vi "AcurrDataIn.vi"(0 "AMP":dbl, 1 "Max":dbl, 2 "Period":dbl, 3 "通道":u16(ring) items=["CH1", "CH2", "CH3", "CH4", "CH5", "CH6", "CH7", "CH8", "CH9", "CH10"], 5 "RMS":dbl, 7 "Min":dbl, 9 "Vpkpk":dbl, 11 "error in (no error)":errorcluster, 12 "FREQ":dbl, 13 "温度":dbl, 14 "测试类型":string) -> (15 "error out":errorcluster)   [LabVIEW 2014]
uses:
  <vilib>/addons/database/Connection.llb/DB Tools Open Connec (String).vi
  <vilib>/addons/database/Connection.llb/Conn Execute.vi
  <vilib>/addons/database/Recordset.llb/Rec Destroy - Connection.vi
  <vilib>/addons/database/NI_Database_API.lvlib
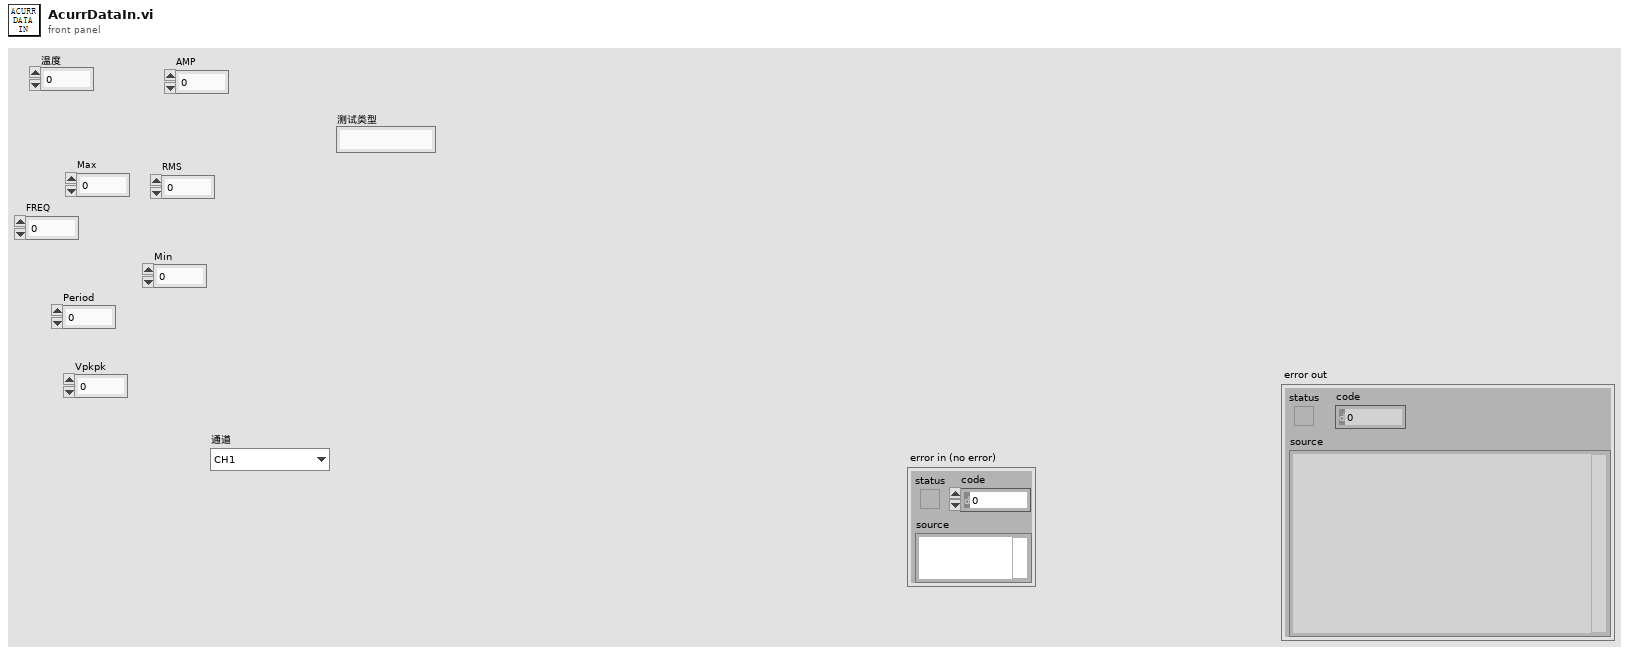
[diagram p1: front panel]
types:
  T1 = typedef "NI_Database_API.lvlib/Conn ObjectReference.ctl" = refnum<k1>
  T2 = typedef "NI_Database_API.lvlib/Rec ObjectReference.ctl" = refnum<k1>
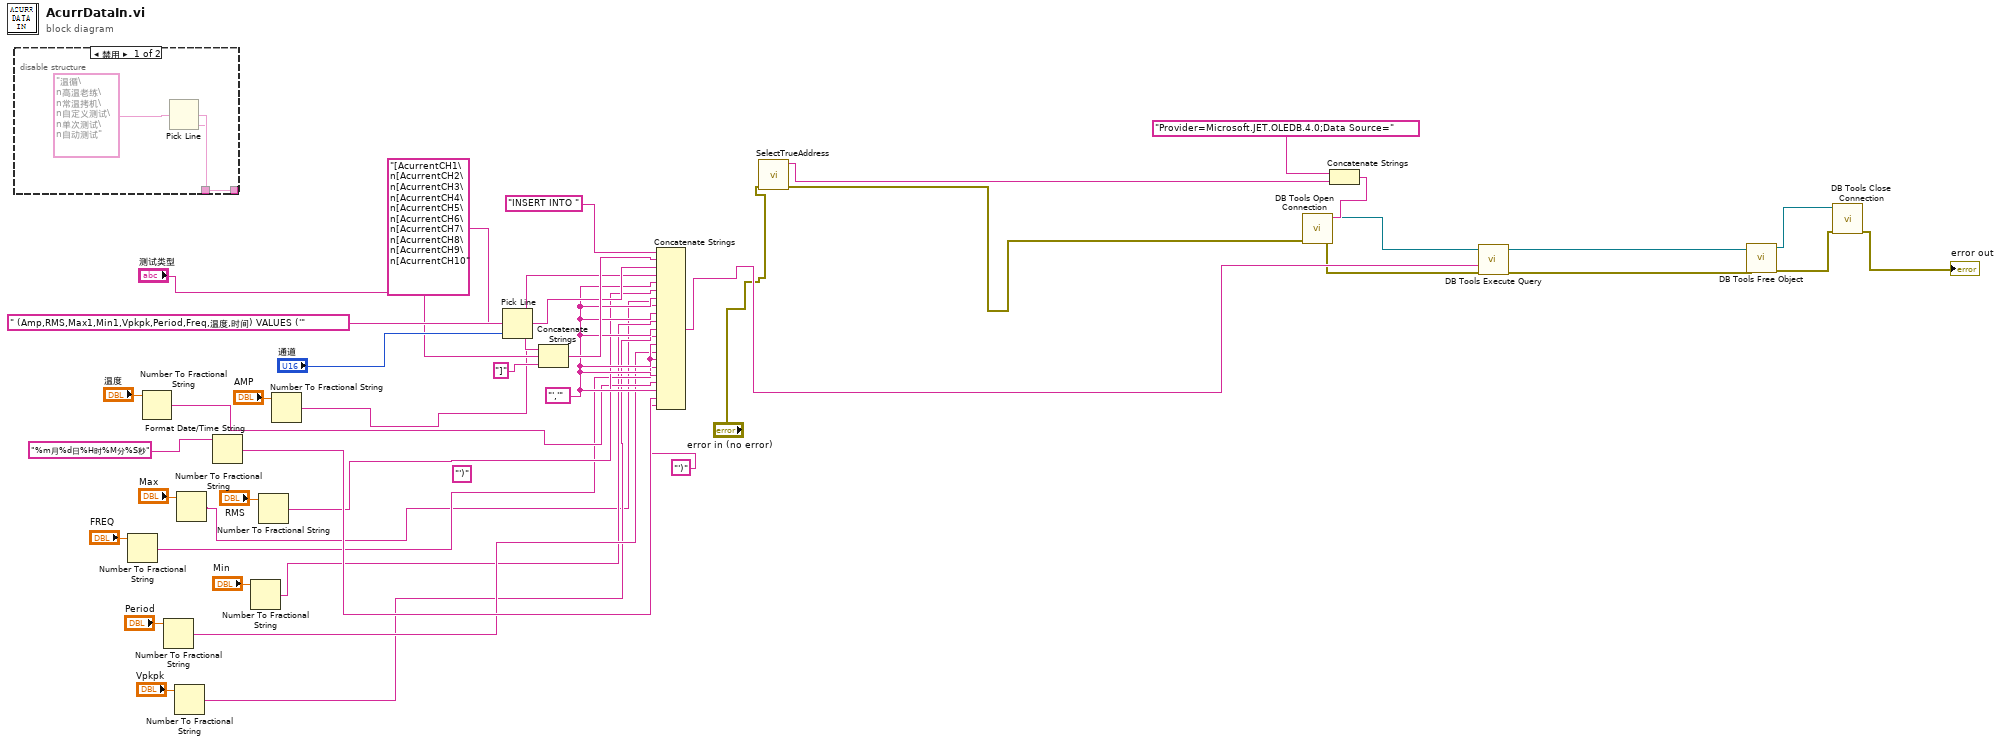
[diagram p0: block diagram]
diagram:
  w34 = "','"
  (unwired) "')"
  n1 = disable-structure shown="禁用" {
    disable-tunnel: [w44 _] -> _
    disable-tunnel: _ -> [w43 _]
    frame Disabled {
      n2 = Pick Line(multi-line string="温循\n高温老练\n常温拷机\n自定义测试\n单次测试\n自动测试" ("多行字符串"), line index=w43) -> (output string=w44:string)  [unwired: 1 in]
    }
    frame Enabled {
    }
  }
  n3 = Number To Fractional String(number="FREQ") -> (F-format string=w22:string)  [unwired: 3 in]
  n4 = Number To Fractional String(number="温度") -> (F-format string=w24:string)  [unwired: 3 in]
  n5 = Number To Fractional String(number="Period") -> (F-format string=w20:string)  [unwired: 3 in]
  n6 = Number To Fractional String(number="Vpkpk") -> (F-format string=w18:string)  [unwired: 3 in]
  n7 = Number To Fractional String(number="Max") -> (F-format string=w14:string)  [unwired: 3 in]
  n8 = Format Date/Time String(time format string (%c)="%m月%d日%H时%M分%S秒" ("时间格式字符串(%c)")) -> (date/time string=w32:string)  [unwired: 2 in]
  n9 = Number To Fractional String(number="Min") -> (F-format string=w16:string)  [unwired: 3 in]
  n10 = Number To Fractional String(number="RMS") -> (F-format string=w26:string)  [unwired: 3 in]
  n11 = Number To Fractional String(number="AMP") -> (F-format string=w29:string)  [unwired: 3 in]
  n12 = Pick Line(multi-line string="[AcurrentCH1\n[AcurrentCH2\n[AcurrentCH3\n[AcurrentCH4\n[AcurrentCH5\n[AcurrentCH6\n[AcurrentCH7\n[AcurrentCH8\n[AcurrentCH9\n[AcurrentCH10" ("多行字符串"), line index="通道") -> (output string=w40:string)  [unwired: 1 in]
  n13 = Concatenate Strings(w40, "测试类型", "]") -> (w39:string)
  n14 = Concatenate Strings("INSERT INTO ", w39, " (Amp,RMS,Max1,Min1,Vpkpk,Period,Freq,温度,时间) VALUES ('", w29, w34, w26, w34, w14, w34, w16, w34, w18, w34, w20, w34, w22, w34, w24, w34, w32, "')") -> (w12:string)
  n15 = call "SelectTrueAddress.vi"("error in (no error)"="error in (no error)") -> ("error out"=w1:errorcluster, "元素"=w13:string)  [unwired: 9 in]
  n16 = Concatenate Strings("Provider=Microsoft.JET.OLEDB.4.0;Data Source=", w13) -> (w9:string)
  n17 = call-poly <vilib>:"DB Tools Open Connection.vi"("error in (no error)"=w1, "connection information"=w9) -> ("error out"=w7:errorcluster, "connection reference"=w8:T1)  [unwired: 6 in]
  n18 = call-poly <vilib>:"DB Tools Execute Query.vi"("error in (no error)"=w7, "SQL query"=w12, "connection reference"=w8) -> ("error out"=w5:errorcluster, "recordset reference"=w6:T2)  [unwired: 5 in]
  n19 = call-poly <vilib>:"DB Tools Free Object.vi"("error in (no error)"=w5, "recordset reference"=w6) -> ("error out"=w3:errorcluster, "connection reference"=w4:T1)  [unwired: 8 in]
  n20 = call <vilib>:"DB Tools Close Connection.vi"("error in (no error)"=w3, "connection reference"=w4) -> ("error out"=→"error out":errorcluster)  [unwired: 5 in]
